vi "MessageService.vi"(8 "error in (no error)":errorcluster, 10 "Message":string, 11 "Service Name":string) -> (0 "error out":errorcluster, 3 "Response":string)   [LabVIEW 2019, in "MicronManager.lvclass"]
uses:
  MicronManager.lvclass
  <vilib>/SLL Toolkit/SLL Easy TCP/_SubVIs/TCP Initialize Client - Local.vi
  <vilib>/SLL Toolkit/SLL Easy TCP/SLL Easy API via TCP.lvclass
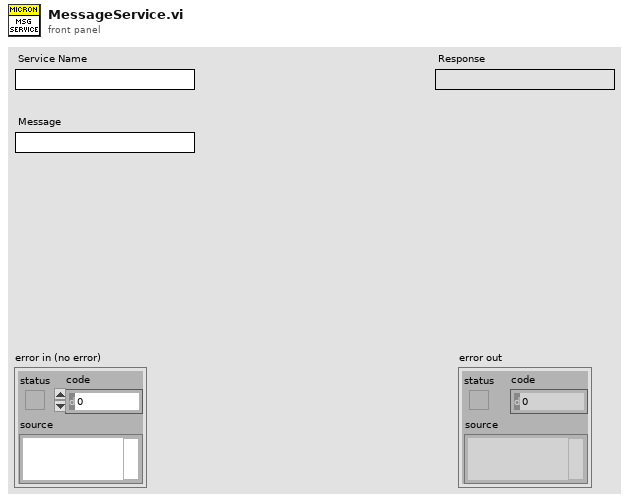
[diagram p1: front panel]
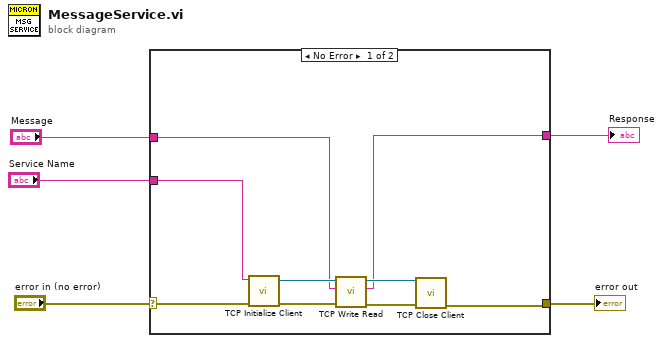
[diagram p0: block diagram]
diagram:
  n1 = case shown="No Error" "error in (no error)" {
    selector: "error in (no error)" -> [w10 w15]
    tunnel: [w9 w15] -> w4
    tunnel: "Message" -> [w7 _]
    tunnel: "Service Name" -> [w8 _]
    tunnel: [w6 _] -> w1
    frame No Error {
      n2 = call-poly <vilib>:"TCP Initialize Client.vi"("error in (no error)"=w10, "Service Name"=w8) -> ("error out"=w13:errorcluster, "connection ID Out"=w11:refnum<k5>)  [unwired: 8 in]
      n3 = call <vilib>:"TCP Write Read.vi"("error in (no error)"=w13, "Write Data"=w7, "connection ID In"=w11) -> ("error out"=w14:errorcluster, "Read Data"=w6:string, "connection ID Out"=w12:refnum<k5>)  [unwired: 5 in, 1 out]
      n4 = call <vilib>:"TCP Close Client.vi"("error in (no error)"=w14, "connection ID"=w12) -> ("error out"=w9:errorcluster)  [unwired: 9 in]
    }
    frame Error {
    }
  }
  "error out" <- w4
  "Response" <- w1
